vi "Search.vi"(7 "Parent ID":string, 8 "Error In":errorcluster, 10 "Name":string, 11 "Tree Manager":T1) -> (0 "Error Out":errorcluster, 1 "IDs":string[](array[string]), 3 "Tree Manager":T1)   [LabVIEW 2016, in "Tree Manager.lvclass"]
doc: "Search through the Tree Manager to find a Tree with a specific name. \n\nIf the Parent ID is wired the search will be shallow, limited to only the Children of the Parent Tree.\n\nIf the Parent ID is <b>NOT</b> wired a global search will be performed, through all Trees.\n\nThe returned array of IDs contains the IDs of <b>ALL</b> Trees with a matching name."
uses:
  Tree Manager.lvclass
  Typedefs/Session Handle.ctl
  Tree Manager.lvclass/Tree Manager.ctl
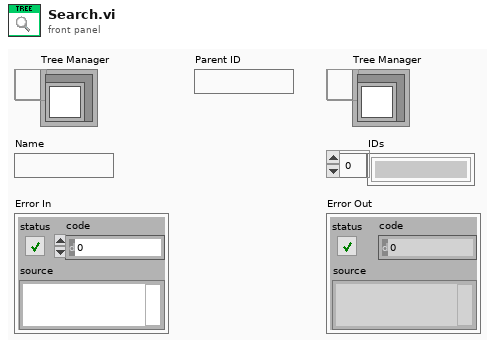
[diagram p1: front panel]
types:
  T1 = typedef "Tree Manager.lvclass/Session Handle.ctl" = refnum<data-value>
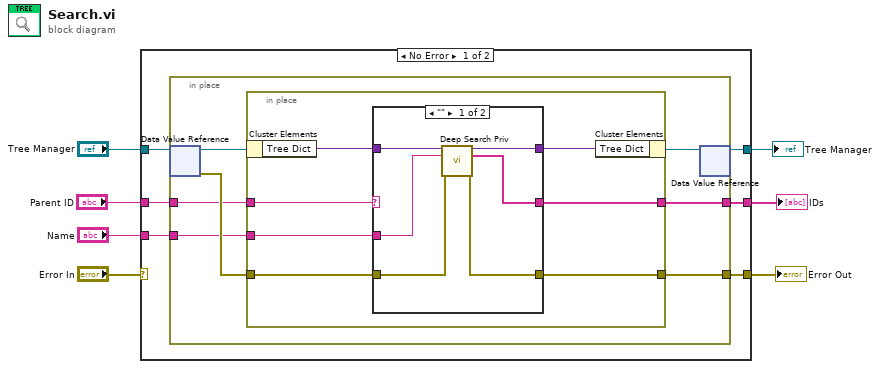
[diagram p0: block diagram]
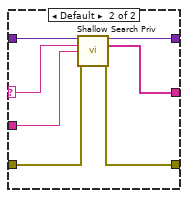
[diagram p2: hidden frame]
diagram:
  n1 = case shown="No Error" "Error In" {
    selector: "Error In" -> [_ w41]
    tunnel: "Tree Manager" -> [w13 w42]
    tunnel: [w12 w42] -> w6
    tunnel: [w11 w41] -> w4
    tunnel: "Parent ID" -> [w10 _]
    tunnel: "Name" -> [w9 _]
    tunnel: [w8 _] -> w1
    frame No Error {
      n2 = in-place {
        in-place-border: [w19] -> w11
        in-place-border: w10 -> [w16]
        in-place-border: w9 -> [w15]
        in-place-border: [w14] -> w8
        n3 = in-place-dvr #1(w13) -> (w20:refnum<class "Tree Manager.lvclass">, w17:errorcluster)
        n4 = in-place {
          in-place-border: [w24] -> w19
          in-place-border: w17 -> [w25]
          in-place-border: w16 -> [w21]
          in-place-border: w15 -> [w23]
          in-place-border: [w22] -> w14
          n5 = in-place-cluster #2(w20) -> ("Tree Dict"=w27:variant)
          n6 = case shown="\"\"" w21 {
            selector: w21 -> [_ w34]
            tunnel: w27 -> [w33 w40]
            tunnel: [w32 w39] -> w26
            tunnel: w25 -> [w29 w38]
            tunnel: [w30 w37] -> w24
            tunnel: w23 -> [w28 w36]
            tunnel: [w31 w35] -> w22
            frame "" {
              n7 = call "Deep Search Priv.vi"("Tree Dictionary In"=w33, "Name"=w28, "error in"=w29) -> ("Tree Dictionary Out"=w32:variant, "IDs"=w31:string[], "error out"=w30:errorcluster)  [unwired: 10 in]
            }
            frame Default {
              n8 = call "Shallow Search Priv.vi"("Tree Dictionary In"=w40, "Unique ID"=w34, "Name"=w36, "error in"=w38) -> ("Tree Dictionary Out"=w39:variant, "IDs"=w35:string[], "error out"=w37:errorcluster)  [unwired: 9 in]
            }
          }
          n9 = in-place-cluster #2("Tree Dict"=w26) -> (w18:refnum<class "Tree Manager.lvclass">)
        }
        n10 = in-place-dvr #1(w18) -> (w12:T1)  [unwired: 1 out]
      }
    }
    frame Error {
    }
  }
  "Tree Manager" <- w6
  "Error Out" <- w4
  "IDs" <- w1
